vi "Shared Variable Units Tests.vi"   [LabVIEW 2021]
uses:
  Source/DBL/conc_SharedVar_DBL.lvclass
  <vilib>/TSA/Abstract Data Classes/Abs_Types/Double Float/Abs_Double Float.lvclass
  C:/Program Files (x86)/National Instruments/LabVIEW 2021/vi.lib/TSA/Abstract Data Classes/Abs_Types/Type/Abs_Type.lvclass
  <vilib>/TSA/Abstract Data Classes/Abs_Types/Single Float/Abs_Single Float.lvclass
  Source/SGL/conc_SharedVar_SGL.lvclass
  Source/I8/conc_SharedVar_I8.lvclass
  <vilib>/TSA/Abstract Data Classes/Abs_Types/I8 Integer/Abs_I8 Integer.lvclass
  <vilib>/TSA/Abstract Data Classes/Abs_Types/I16 Integer/Abs_I16 Integer.lvclass
  Source/I16/conc_SharedVar_I16.lvclass
  Source/I32/conc_SharedVar_I32.lvclass
  <vilib>/TSA/Abstract Data Classes/Abs_Types/I32 Integer/Abs_I32 Integer.lvclass
  <vilib>/TSA/Abstract Data Classes/Abs_Types/I64 Integer/Abs_I64 Integer.lvclass
  Source/I64/conc_SharedVar_I64.lvclass
  <vilib>/TSA/Abstract Data Classes/Abs_Types/U8 Integer/Abs_U8 Integer.lvclass
  <vilib>/TSA/Abstract Data Classes/Abs_Types/U16 Integer/Abs_U16 Integer.lvclass
  <vilib>/TSA/Abstract Data Classes/Abs_Types/U32 Integer/Abs_U32 Integer.lvclass
  <vilib>/TSA/Abstract Data Classes/Abs_Types/U64 Integer/Abs_U64 Integer.lvclass
  Source/U8/conc_SharedVar_U8.lvclass
  Source/U16/conc_SharedVar_U16.lvclass
  Source/U32/conc_SharedVar_U32.lvclass
  Source/U64/conc_SharedVar_U64.lvclass
  278aed17-6c92-49f2-9fb8-5e9110347083.vi
  49a8c154-cbd4-4358-857c-2782e17b93d6.vi
  00fedc10-3c52-4491-a0d0-45cf9733179c.vi
  4f70bbd9-0e16-4429-94fe-751a44574fc1.vi
  192ef0b5-e00d-4ad6-a6c0-7e0975484183.vi
  ddf351a1-fe68-4aed-bc64-f160ec6d45ca.vi
  ba9fb781-2b88-423f-aed2-93569e1d02dc.vi
  64901ce4-aebb-4275-af15-a99de37dfb3a.vi
  d119a695-ff97-4b64-8931-cabbc027a1d7.vi
  b7af582b-8ca9-4fb0-bc3b-f76cc04d0d41.vi
  278aed17-6c92-49f2-9fb8-5e9110347083.vi/9c5f5204-69d5-44b0-9fed-84ac97b71057.vi
  278aed17-6c92-49f2-9fb8-5e9110347083.vi/103af6e5-0f20-4bd9-87ce-4bacf20ebd2f.vi
  49a8c154-cbd4-4358-857c-2782e17b93d6.vi/9c5f5204-69d5-44b0-9fed-84ac97b71057.vi
  49a8c154-cbd4-4358-857c-2782e17b93d6.vi/103af6e5-0f20-4bd9-87ce-4bacf20ebd2f.vi
  00fedc10-3c52-4491-a0d0-45cf9733179c.vi/9c5f5204-69d5-44b0-9fed-84ac97b71057.vi
  00fedc10-3c52-4491-a0d0-45cf9733179c.vi/103af6e5-0f20-4bd9-87ce-4bacf20ebd2f.vi
  4f70bbd9-0e16-4429-94fe-751a44574fc1.vi/9c5f5204-69d5-44b0-9fed-84ac97b71057.vi
  4f70bbd9-0e16-4429-94fe-751a44574fc1.vi/103af6e5-0f20-4bd9-87ce-4bacf20ebd2f.vi
  192ef0b5-e00d-4ad6-a6c0-7e0975484183.vi/9c5f5204-69d5-44b0-9fed-84ac97b71057.vi
  192ef0b5-e00d-4ad6-a6c0-7e0975484183.vi/103af6e5-0f20-4bd9-87ce-4bacf20ebd2f.vi
  ddf351a1-fe68-4aed-bc64-f160ec6d45ca.vi/9c5f5204-69d5-44b0-9fed-84ac97b71057.vi
  ddf351a1-fe68-4aed-bc64-f160ec6d45ca.vi/103af6e5-0f20-4bd9-87ce-4bacf20ebd2f.vi
  ba9fb781-2b88-423f-aed2-93569e1d02dc.vi/9c5f5204-69d5-44b0-9fed-84ac97b71057.vi
  ba9fb781-2b88-423f-aed2-93569e1d02dc.vi/103af6e5-0f20-4bd9-87ce-4bacf20ebd2f.vi
  64901ce4-aebb-4275-af15-a99de37dfb3a.vi/9c5f5204-69d5-44b0-9fed-84ac97b71057.vi
  64901ce4-aebb-4275-af15-a99de37dfb3a.vi/103af6e5-0f20-4bd9-87ce-4bacf20ebd2f.vi
  d119a695-ff97-4b64-8931-cabbc027a1d7.vi/9c5f5204-69d5-44b0-9fed-84ac97b71057.vi
  d119a695-ff97-4b64-8931-cabbc027a1d7.vi/103af6e5-0f20-4bd9-87ce-4bacf20ebd2f.vi
  b7af582b-8ca9-4fb0-bc3b-f76cc04d0d41.vi/9c5f5204-69d5-44b0-9fed-84ac97b71057.vi
  b7af582b-8ca9-4fb0-bc3b-f76cc04d0d41.vi/103af6e5-0f20-4bd9-87ce-4bacf20ebd2f.vi
  Support/String shared Variable Test.vi/9c5f5204-69d5-44b0-9fed-84ac97b71057.vi
  Support/String shared Variable Test.vi/103af6e5-0f20-4bd9-87ce-4bacf20ebd2f.vi
  Support/Bool shared Variable Test.vi/9c5f5204-69d5-44b0-9fed-84ac97b71057.vi
  Support/Bool shared Variable Test.vi/103af6e5-0f20-4bd9-87ce-4bacf20ebd2f.vi
  Support/Variant shared Variable Test.vi/9c5f5204-69d5-44b0-9fed-84ac97b71057.vi
  Support/Variant shared Variable Test.vi/103af6e5-0f20-4bd9-87ce-4bacf20ebd2f.vi
  Support/WFM shared Variable Test.vi/9c5f5204-69d5-44b0-9fed-84ac97b71057.vi
  Support/WFM shared Variable Test.vi/103af6e5-0f20-4bd9-87ce-4bacf20ebd2f.vi
  <vilib>/TSA/Abstract Data Classes/Abs_Types/String/Abs_String.lvclass
  <vilib>/TSA/Abstract Data Classes/Abs_Types/Boolean/Abs_Boolean.lvclass
  <vilib>/TSA/Abstract Data Classes/Abs_Types/Variant/Abs_Variant.lvclass
  <vilib>/TSA/Abstract Data Classes/Abs_Types/Waveform/Abs_Waveform.lvclass
  <vilib>/Utility/Data Type/Get Type Information.vi
  <vilib>/addons/_JKI Toolkits/Caraya/classes/Test/Define Test.vi
  <vilib>/TSA/Abstract Data Classes/Abs_Types/Type/Read Config JSON.vi
  <vilib>/TSA/Abstract Data Classes/Abs_Types/Abs_Read.vi
  <vilib>/TSA/Abstract Data Classes/Abs_Types/Double Float/Static Read.vi
  <vilib>/addons/_JKI Toolkits/Caraya/classes/Assert/Assert.vi
  <vilib>/addons/_JKI Toolkits/Caraya/classes/Assert/Assert Almost Equal_Float.vi
  <vilib>/addons/_JKI Toolkits/Caraya/classes/Assert/Assert Equal Type_Variant.vi
  <vilib>/TSA/Abstract Data Classes/Abs_Types/Abs_Write.vi
  <vilib>/TSA/Abstract Data Classes/Abs_Types/Double Float/Static Write.vi
  <vilib>/TSA/Abstract Data Classes/Abs_Types/Single Float/Static Read.vi
  <vilib>/TSA/Abstract Data Classes/Abs_Types/Single Float/Static Write.vi
  <vilib>/TSA/Abstract Data Classes/Abs_Types/I8 Integer/Static Read.vi
  <vilib>/TSA/Abstract Data Classes/Abs_Types/I8 Integer/Static Write.vi
  <vilib>/TSA/Abstract Data Classes/Abs_Types/I16 Integer/Static Read.vi
  <vilib>/TSA/Abstract Data Classes/Abs_Types/I16 Integer/Static Write.vi
  <vilib>/TSA/Abstract Data Classes/Abs_Types/I32 Integer/Static Read.vi
  <vilib>/TSA/Abstract Data Classes/Abs_Types/I32 Integer/Static Write.vi
  <vilib>/TSA/Abstract Data Classes/Abs_Types/I64 Integer/Static Read.vi
  <vilib>/TSA/Abstract Data Classes/Abs_Types/I64 Integer/Static Write.vi
  <vilib>/TSA/Abstract Data Classes/Abs_Types/U8 Integer/Static Read.vi
  <vilib>/TSA/Abstract Data Classes/Abs_Types/U8 Integer/Static Write.vi
  <vilib>/TSA/Abstract Data Classes/Abs_Types/U16 Integer/Static Read.vi
  <vilib>/TSA/Abstract Data Classes/Abs_Types/U16 Integer/Static Write.vi
  <vilib>/TSA/Abstract Data Classes/Abs_Types/U32 Integer/Static Read.vi
  <vilib>/TSA/Abstract Data Classes/Abs_Types/U32 Integer/Static Write.vi
  <vilib>/TSA/Abstract Data Classes/Abs_Types/U64 Integer/Static Read.vi
  <vilib>/TSA/Abstract Data Classes/Abs_Types/U64 Integer/Static Write.vi
  <vilib>/TSA/Abstract Data Classes/Abs_Types/String/Static Read.vi
  <vilib>/addons/_JKI Toolkits/Caraya/classes/Assert/Assert Equal Value_Variant.vi
  <vilib>/TSA/Abstract Data Classes/Abs_Types/String/Static Write.vi
  <vilib>/TSA/Abstract Data Classes/Abs_Types/Boolean/Static Read.vi
  <vilib>/TSA/Abstract Data Classes/Abs_Types/Boolean/Static Write.vi
  <vilib>/TSA/Abstract Data Classes/Abs_Types/Variant/Static Read.vi
  <vilib>/TSA/Abstract Data Classes/Abs_Types/Variant/Static Write.vi
  <vilib>/TSA/Abstract Data Classes/Abs_Types/Waveform/Static Read.vi
  <vilib>/TSA/Abstract Data Classes/Abs_Types/Waveform/Static Write.vi
  Source/STR/conc_SharedVar_STR.lvclass
  Source/Bool/conc_SharedVar_Bool.lvclass
  Source/Var/conc_SharedVar_Var.lvclass
  Source/WFM/conc_SharedVar_WFM.lvclass
  <vilib>/measure/NI_MABase.lvlib
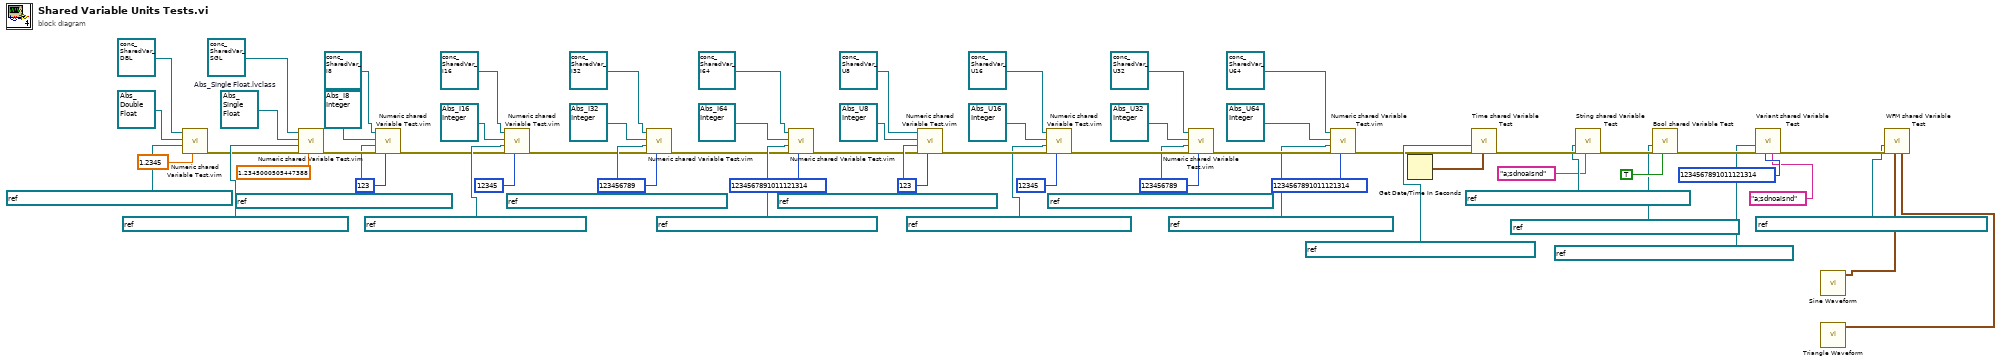
[diagram p0: block diagram]
diagram:
  w60 = refnum<class "Abs_Single Float.lvclass"> refnum  # Abs_Single Float.lvclass
  n1 = call "Numeric shared Variable Test.vim"("Value"=1.2345, "shared variable refnum"=refnum<k21> "ni.var.psp://localhost/Test Shared Variables/DBL", "Abs_Single Float.lvclass"=refnum<class "Abs_Double Float.lvclass"> refnum ("Abs_Double Float.lvclass"), "abs_SharedVar_Class"=refnum<class "conc_SharedVar_DBL.lvclass"> refnum) -> ("error out"=w59:errorcluster)  [unwired: 7 in]
  n2 = call "Numeric shared Variable Test.vim"("Value"=sgl 1.2345, "error in (no error)"=w59, "shared variable refnum"=refnum<k21> "ni.var.psp://localhost/Test Shared Variables/SGL", "Abs_Single Float.lvclass"=w60, "abs_SharedVar_Class"=refnum<class "conc_SharedVar_SGL.lvclass"> refnum ("conc_SharedVar_SGL.lvclass")) -> ("error out"=w57:errorcluster)  [unwired: 6 in]
  n3 = call "Numeric shared Variable Test.vim"("Value"=i8 123, "error in (no error)"=w57, "shared variable refnum"=refnum<k21> "ni.var.psp://localhost/Test Shared Variables/I8", "Abs_Single Float.lvclass"=refnum<class "Abs_I8 Integer.lvclass"> refnum ("Abs_I8 Integer.lvclass"), "abs_SharedVar_Class"=refnum<class "conc_SharedVar_I8.lvclass"> refnum ("conc_SharedVar_I8.lvclass")) -> ("error out"=w50:errorcluster)  [unwired: 6 in]
  n4 = call "Numeric shared Variable Test.vim"("Value"=i16 12345, "error in (no error)"=w50, "shared variable refnum"=refnum<k21> "ni.var.psp://localhost/Test Shared Variables/I16", "Abs_Single Float.lvclass"=refnum<class "Abs_I16 Integer.lvclass"> refnum ("Abs_I16 Integer.lvclass"), "abs_SharedVar_Class"=refnum<class "conc_SharedVar_I16.lvclass"> refnum ("conc_SharedVar_I16.lvclass")) -> ("error out"=w45:errorcluster)  [unwired: 6 in]
  n5 = call "Numeric shared Variable Test.vim"("Value"=123456789, "error in (no error)"=w45, "shared variable refnum"=refnum<k21> "ni.var.psp://localhost/Test Shared Variables/I32", "Abs_Single Float.lvclass"=refnum<class "Abs_I32 Integer.lvclass"> refnum ("Abs_I32 Integer.lvclass"), "abs_SharedVar_Class"=refnum<class "conc_SharedVar_I32.lvclass"> refnum ("conc_SharedVar_I32.lvclass")) -> ("error out"=w40:errorcluster)  [unwired: 6 in]
  n6 = call "Numeric shared Variable Test.vim"("Value"=i64 1234567891011121314, "error in (no error)"=w40, "shared variable refnum"=refnum<k21> "ni.var.psp://localhost/Test Shared Variables/I64", "Abs_Single Float.lvclass"=refnum<class "Abs_I64 Integer.lvclass"> refnum ("Abs_I64 Integer.lvclass"), "abs_SharedVar_Class"=refnum<class "conc_SharedVar_I64.lvclass"> refnum ("conc_SharedVar_I64.lvclass")) -> ("error out"=w26:errorcluster)  [unwired: 6 in]
  n7 = call "Numeric shared Variable Test.vim"("Value"=u8 123, "error in (no error)"=w26, "shared variable refnum"=refnum<k21> "ni.var.psp://localhost/Test Shared Variables/U8", "Abs_Single Float.lvclass"=refnum<class "Abs_U8 Integer.lvclass"> refnum ("Abs_U8 Integer.lvclass"), "abs_SharedVar_Class"=refnum<class "conc_SharedVar_U8.lvclass"> refnum ("conc_SharedVar_U8.lvclass")) -> ("error out"=w31:errorcluster)  [unwired: 6 in]
  n8 = call "Numeric shared Variable Test.vim"("Value"=u16 12345, "error in (no error)"=w31, "shared variable refnum"=refnum<k21> "ni.var.psp://localhost/Test Shared Variables/U16", "Abs_Single Float.lvclass"=refnum<class "Abs_U16 Integer.lvclass"> refnum ("Abs_U16 Integer.lvclass"), "abs_SharedVar_Class"=refnum<class "conc_SharedVar_U16.lvclass"> refnum ("conc_SharedVar_U16.lvclass")) -> ("error out"=w34:errorcluster)  [unwired: 6 in]
  n9 = call "Numeric shared Variable Test.vim"("Value"=u32 123456789, "error in (no error)"=w34, "shared variable refnum"=refnum<k21> "ni.var.psp://localhost/Test Shared Variables/U32", "Abs_Single Float.lvclass"=refnum<class "Abs_U32 Integer.lvclass"> refnum ("Abs_U32 Integer.lvclass"), "abs_SharedVar_Class"=refnum<class "conc_SharedVar_U32.lvclass"> refnum ("conc_SharedVar_U32.lvclass")) -> ("error out"=w37:errorcluster)  [unwired: 6 in]
  n10 = call "Numeric shared Variable Test.vim"("Value"=u64 1234567891011121314, "error in (no error)"=w37, "shared variable refnum"=refnum<k21> "ni.var.psp://localhost/Test Shared Variables/U64", "Abs_Single Float.lvclass"=refnum<class "Abs_U64 Integer.lvclass"> refnum ("Abs_U64 Integer.lvclass"), "abs_SharedVar_Class"=refnum<class "conc_SharedVar_U64.lvclass"> refnum ("conc_SharedVar_U64.lvclass")) -> ("error out"=w12:errorcluster)  [unwired: 6 in]
  n11 = Get Date/Time In Seconds() -> (seconds since 1Jan1904=w16:timestamp)
  n12 = call "Time shared Variable Test.vi"("Value"=w16, "error in (no error)"=w12, "shared variable refnum"=refnum<k21> "ni.var.psp://localhost/Test Shared Variables/Time") -> ("error out"=w15:errorcluster)  [unwired: 8 in]
  n13 = call "String shared Variable Test.vi"("Value"="a;sdnoaisnd", "error in (no error)"=w15, "shared variable refnum"=refnum<k21> "ni.var.psp://localhost/Test Shared Variables/STR") -> ("error out"=w11:errorcluster)  [unwired: 8 in]
  n14 = call "Bool shared Variable Test.vi"("Value"=TRUE, "error in (no error)"=w11, "shared variable refnum"=refnum<k21> "ni.var.psp://localhost/Test Shared Variables/Bool") -> ("error out"=w8:errorcluster)  [unwired: 8 in]
  n15 = call "Variant shared Variable Test.vi"("Value 2"="a;sdnoaisnd" ("Value"), "Value"=u64 1234567891011121314, "error in (no error)"=w8, "shared variable refnum"=refnum<k21> "ni.var.psp://localhost/Test Shared Variables/Variant") -> ("error out"=w4:errorcluster)  [unwired: 7 in]
  n16 = call <vilib>:"Sine Waveform.vi"() -> ("signal out"=w2:waveform(dbl))  [unwired: 10 in, 1 out]
  n17 = call <vilib>:"Triangle Waveform.vi"() -> ("signal out"=w1:waveform(dbl))  [unwired: 10 in, 1 out]
  n18 = call "WFM shared Variable Test.vi"("Waveform 2"=w1, "Waveform"=w2, "error in (no error)"=w4, "shared variable refnum"=refnum<k21> "ni.var.psp://localhost/Test Shared Variables/WFM") -> ()  [unwired: 7 in, 1 out]
